vi "Equi-Ripple LowPass PtByPt.vi"(4 "initialize":bool, 5 "stop freq":dbl=0.25 format="%0.2f", 6 "pass freq":dbl=0.2 format="%0.2f", 7 "# of taps":i32=32, 9 "sampling freq: fs":dbl=1.0 format="%0.2f", 10 "x":dbl format="%0.2f") -> (0 "error":i32, 3 "Filtered x":dbl format="%0.2f")   [LabVIEW 2020, in "NI_PtbyPt.lvlib"]
doc: "Filters <B>x</B> using an equi-ripple lowpass FIR filter model."
uses:
  NI_PtbyPt.lvlib
  NI_AALBase.lvlib
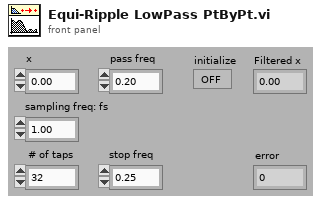
[diagram p1: front panel]
types:
  T1 = cluster{"Amplitude":dbl, "DC":dbl, "pass freq":dbl, "Weight":dbl}
  T2 = cluster{"Amplitude":dbl, "stop freq":dbl, dbl, "Weight":dbl}
  T3 = cluster{"Amplitude":dbl, "stop freq":dbl, "pass freq":dbl, "Weight":dbl}[]
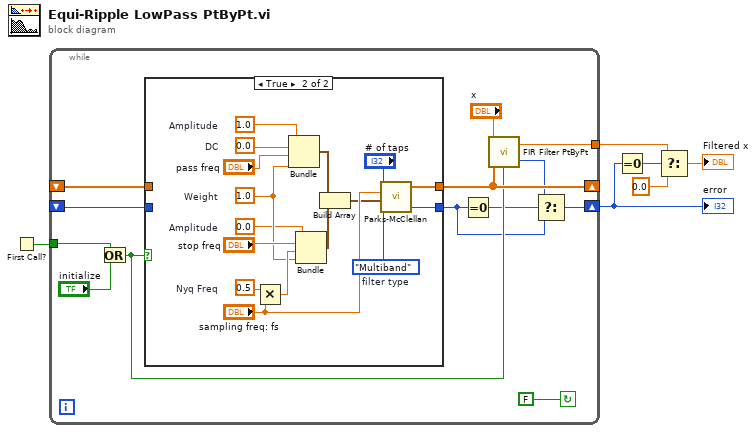
[diagram p0: block diagram]
diagram:
  n1 = First Call?() -> (First Call?: T/F=w6:bool)
  n2 = while {
    tunnel: w6 -> [w15]
    shift-left: _ -> [w19]
    shift-right: [w18] -> _
    shift-right: [w9] -> w5
    shift-left: _ -> [w8]
    tunnel: [w7] -> w3
    stop <- FALSE continue-if-true
    n3 = Or(x=w15, y="initialize") -> (x .or. y?=w13:bool)
    n4 = case shown="True" w13 {
      tunnel: [w21 w37] -> w18
      tunnel: w19 -> [w21 _]
      tunnel: [w20 w22] -> w10
      tunnel: w8 -> [w20 _]
      frame False {
      }
      frame True {
        w23 = enum32{"Multiband", "Differentiator", "Hilbert"}."Multiband"  # filter type
        w33 = 0.5  # Nyq Freq
        w24 = 0.0  # Amplitude
        w25 = 1.0  # Weight
        w36 = 0.0  # DC
        w26 = 1.0  # Amplitude
        n5 = Multiply(x=w33, y="sampling freq: fs") -> (x*y=w32:dbl)
        n6 = Bundle("Amplitude"=w26, "DC"=w36, "pass freq"="pass freq", "Weight"=w25) -> (w31:T1)  [unwired: 1 out]
        n7 = Bundle("Amplitude"=w24, "stop freq"="stop freq", w32, "Weight"=w25) -> (w30:T2)  [unwired: 1 out]
        n8 = Build Array(w31, w30) -> (w27:T3)
        n9 = call "Parks-McClellan.vi"("filter type"=w23, "Band Parameters"=w27, "sampling freq: fs"="sampling freq: fs", "# of taps"="# of taps") -> ("error"=w22:i32, "h"=w37:dbl[])  [unwired: 1 out]
      }
    }
    n10 = Equal To 0?(x=w10) -> (x = 0?=w12:bool)
    n11 = call "FIR Filter PtByPt.vi"("initialize"=w13, "Forward Coefficients"=w18, "x"="x") -> ("error"=w11:i32, "Filtered x"=w7:dbl)  [unwired: 1 out]
    n12 = Select(t=w11, s=w12, f=w10) -> (s? t:f=w9:i32)
  }
  "error" <- w5
  n13 = Equal To 0?(x=w5) -> (x = 0?=w4:bool)
  n14 = Select(t=w3, s=w4, f=0.0) -> (s? t:f=→"Filtered x":dbl)
